vi "Analog to Digital.vi"   [LabVIEW 2020]
doc: "Converts <B>analog waveform</B> to a digital waveform or digital data. You must manually select the polymorphic instance you want to use."
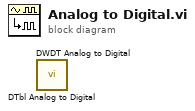
[diagram p0: block diagram]
diagram:
  n1 = call "DTbl Analog to Digital.vi"() -> ()  [unwired: 8 in, 4 out]
  n2 = call "DWDT Analog to Digital.vi"() -> ()  [unwired: 8 in, 4 out]
